vi "read_log_path.vi"(8 "error in (no error)":errorcluster, 11 "data_logger in":refnum<class "data_logger.lvclass">) -> (0 "error out":errorcluster, 2 "log_path":path, 3 "data_logger out":refnum<class "data_logger.lvclass">)   [LabVIEW 2015, in "data_logger.lvclass"]
uses:
  data_logger.lvclass
  data_logger.lvclass/data_logger.ctl
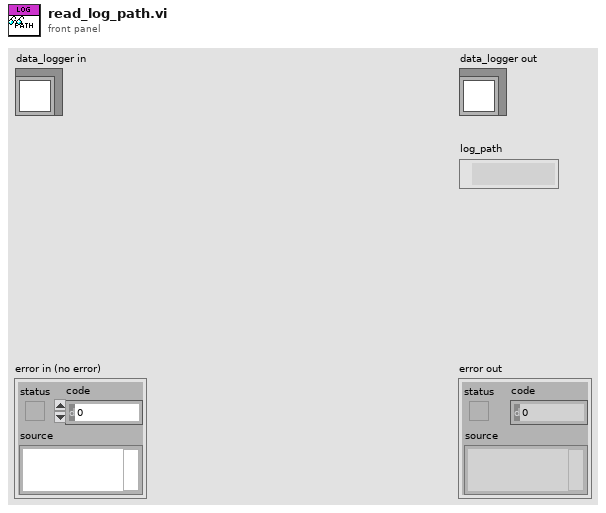
[diagram p1: front panel]
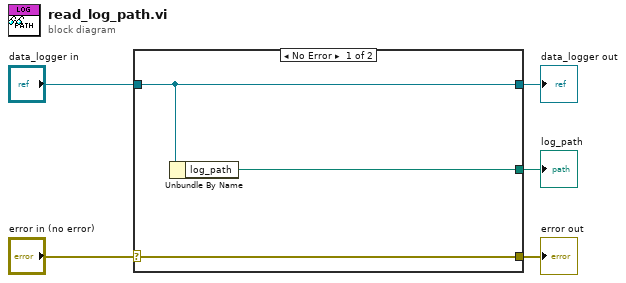
[diagram p0: block diagram]
diagram:
  n1 = case shown="No Error" "error in (no error)" {
    selector: "error in (no error)" -> [w8 w9]
    tunnel: [w8 w9] -> w4
    tunnel: [w7 w10] -> w2
    tunnel: "data_logger in" -> [w7 w10]
    tunnel: [w6 _] -> w1
    frame No Error {
      n2 = Unbundle By Name(w7) -> ("log_path"=w6:path)
    }
    frame Error {
    }
  }
  "error out" <- w4
  "data_logger out" <- w2
  "log_path" <- w1
